vi "Add String.vi"(10 "y":string, 11 "x":string) -> (3 "x + y":string)   [LabVIEW 2013, in "Problem 20.lvlib"]
uses:
  Problem 20.lvlib
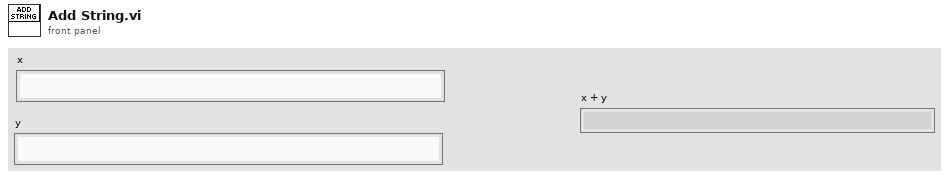
[diagram p1: front panel]
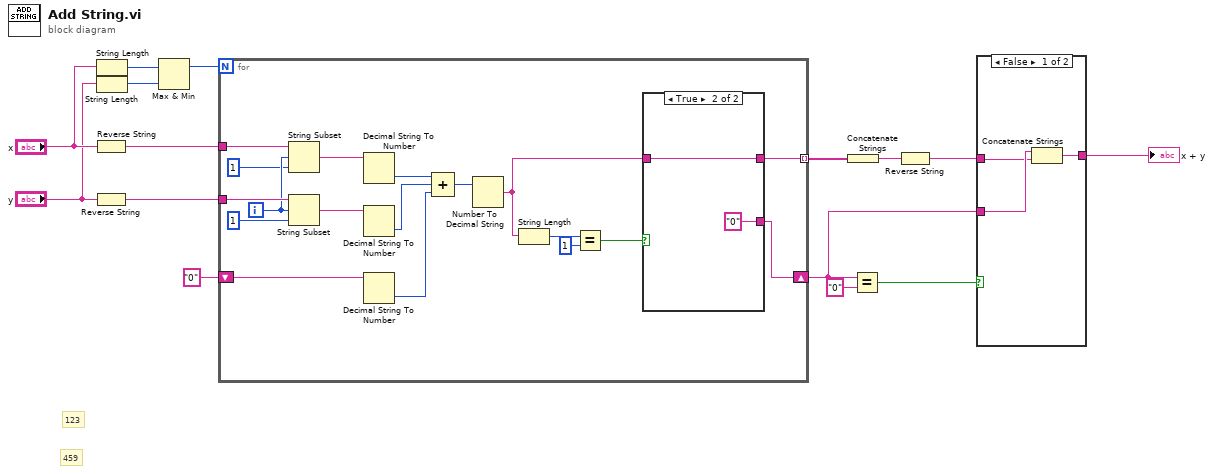
[diagram p0: block diagram]
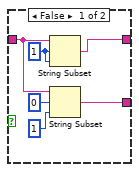
[diagram p3: hidden frame]
diagram:
  # "459"
  # "123"
  n1 = Reverse String(1:"x") -> (0:w10:string)
  n2 = Reverse String(1:"y") -> (0:w9:string)
  n3 = String Length(string="x") -> (length=w13:i32)
  n4 = String Length(string="y") -> (length=w12:i32)
  n5 = Max & Min(x=w13, y=w12) -> (max(x,y)=w11:i32)  [unwired: 1 out]
  n6 = for {
    N: w11 -> [_]
    tunnel: w10 -> [w33]
    tunnel: w9 -> [w32]
    shift-right: [w16] -> w2
    shift-left: "0" -> [w29]
    tunnel: [w17] -> w6 mode=indexing
    i -> [w28]
    n7 = String Subset(string=w33, offset (0)=w28, length (rest)=1 ("length (rest)")) -> (substring=w31:string)
    n8 = String Subset(string=w32, offset (0)=w28, length (rest)=1 ("length (rest)")) -> (substring=w30:string)
    n9 = Decimal String To Number(string=w31) -> (number=w25:i32)  [unwired: 2 in, 1 out]
    n10 = Decimal String To Number(string=w30) -> (number=w23:i32)  [unwired: 2 in, 1 out]
    n11 = Decimal String To Number(string=w29) -> (number=w24:i32)  [unwired: 2 in, 1 out]
    n12 = Compound Arithmetic op=ADD(w25, w23, w24) -> (w22:i32)
    n13 = Number To Decimal String(number=w22) -> (decimal integer string=w18:string)  [unwired: 1 in]
    n14 = String Length(string=w18) -> (length=w20:i32)
    n15 = Equal?(x=w20, y=1) -> (x = y?=w19:bool)
    n16 = case shown="True" w19 {
      tunnel: w18 -> [w36 w41]
      tunnel: [w34 w41] -> w17
      tunnel: [w37 "0"] -> w16
      frame False {
        w35 = 1 ("offset (0)")
        n17 = String Subset(string=w36, offset (0)=w35, length (rest)=w35) -> (substring=w34:string)
        n18 = String Subset(string=w36, offset (0)=0, length (rest)=1 ("length (rest)")) -> (substring=w37:string)
      }
      frame True {
      }
    }
  }
  n19 = Concatenate Strings(w6) -> (w7:string)
  n20 = Equal?(x=w2, y="0") -> (x = y?=w3:bool)
  n21 = Reverse String(1:w7) -> (0:w4:string)
  n22 = case shown="False" w3 {
    tunnel: [w43 w45] -> w1
    tunnel: w2 -> [w44 _]
    tunnel: w4 -> [w42 w45]
    frame False {
      n23 = Concatenate Strings(w44, w42) -> (w43:string)
    }
    frame True {
    }
  }
  "x + y" <- w1
